vi "SVT UFF58 Write Time Waveform (1 Ch).vi"(0 "file refnum":refnum<k20>, 1 "ID lines (1-3)":T2, 2 "data precision (double-precision:1)":T1=1 items=["single-precision", "double-precision"], 5 "waveform":waveform(dbl)={"t0"=timestamp(0 s since 1904-01-01), "dt"=0.0, "Y"=[]}, 11 "error in (no error)":errorcluster) -> (4 "dup file refnum":refnum<k20>, 6 "function refnum":refnum<k20>, 15 "error out":errorcluster)   [LabVIEW 2017, in "SoundVib_UFF58.lvlib"]
doc: "Writes data to the UFF58 (universal file format) file specified by the <B>file refnum</B> input. This VI also writes the fields in records 1, 2, and 3, <B>ID lines (1-3)</B>. You can write a single time domain waveform, multiple time domain waveforms, a single real frequency spectrum, multiple real frequency spectra, a single complex frequency spectrum, multiple complex frequency spectra, or generic data to a UFF file. If a frequency spectrum is in decibels, this VI converts the spectrum to linear before writing to the UFF58 file. The default instance, SVT UFF58 Write Time Waveform (1 Ch), writes a single time domain waveform to the file specified by the <B>file refnum</B> input. Wire data to the <B>file refnum</B> input to determine the polymorphic instance to use or manually select the instance."
uses:
  <vilib>/addons/Sound and Vibration/svt_UFF58/SoundVib_UFF58.lvlib
  <vilib>/addons/Sound and Vibration/svt_UFF58/subVIs/sv_IDLines123.ctl
  <vilib>/addons/Sound and Vibration/svt_UFF58/subVIs/sv_UFF58 Data Precision.ctl
  <vilib>/addons/Sound and Vibration/svt_UFF58/subVIs/sv_UFF58 Check Data Valid (Time) (1Ch).vi
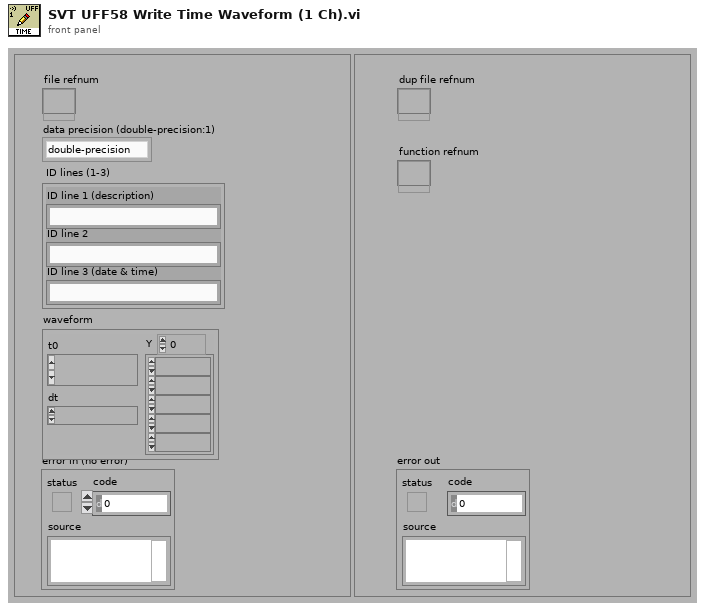
[diagram p1: front panel]
types:
  T1 = typedef "SoundVib_UFF58.lvlib/sv_UFF58 Data Precision.ctl" = u32
  T2 = typedef "SoundVib_UFF58.lvlib/sv_IDLines123.ctl" = cluster{"ID line 1 (description)":string, "ID line 2":string, "ID line 3 (date & time)":string}
  T3 = typedef "SoundVib_UFF58.lvlib/sv_UFF58 DOF.ctl" = cluster{"function type":T4, "function ID number":i32, "version number":i32, "load case ID number":i32, "response entity name":string, "response node":i32, "response direction":T5, "reference entity name":string, "reference node":i32, "reference direction":T5}
  T4 = typedef "SoundVib_UFF58.lvlib/sv_FunctionType.ctl" = enum16{"general or unknown", "time response", "auto spectrum", "cross spectrum", "frequency response function", "transmissibility", "coherence", "auto correlation", "cross correlation", "power spectral density (PSD)", "energy spectral density (ESD)", "probability density function", "spectrum", "cumulative frequency distribution", "peaks valley", "stress/cycles", "strain/cycles", "orbit", "mode indicator function", "force pattern", "partial power", "partial coherence", "eigenvalue", "eigenvector", "shock response spectrum", "finite impulse response filter", "multiple coherence", "order function", "phase compensation"}
  T5 = typedef "SoundVib_UFF58.lvlib/sv_UFF58 Response Direction.ctl" = i32
  T6 = typedef "SoundVib_UFF58.lvlib/sv_UFF58 Axis Characteristics.ctl" = cluster{"specific data type":T7, "length units exponent":i32, "force units exponent":i32, "temperature units exponent":i32, "axis label":string, "axis units label":string}
  T7 = typedef "SoundVib_UFF58.lvlib/sv_UFF58 Specific Datatype.ctl" = u16
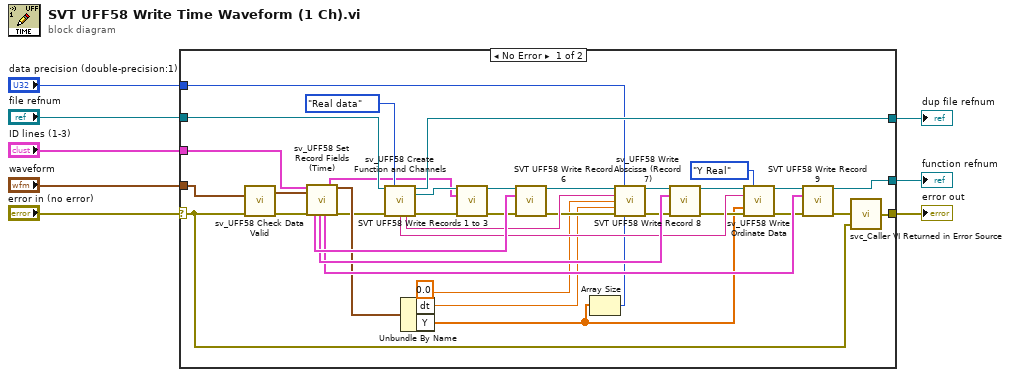
[diagram p0: block diagram]
diagram:
  n1 = case shown="No Error" "error in (no error)" {
    selector: "error in (no error)" -> [w13 w47]
    tunnel: [w14 w47] -> w8
    tunnel: "ID lines (1-3)" -> [w39 _]
    tunnel: [w23 w46] -> w6
    tunnel: "file refnum" -> [w35 w46]
    tunnel: "waveform" -> [w11 _]
    tunnel: [w24 _] -> w2
    tunnel: "data precision (double-precision:1)" -> [w9 _]
    frame No Error {
      n2 = call-poly <vilib>:"sv_UFF58 Check Data Valid.vi"("waveform"=w11, "error in (no error)"=w13) -> ("dup waveform"=w19:waveform(dbl), "error out"=w20:errorcluster)  [unwired: 12 in]
      n3 = call <vilib>:"sv_UFF58 Set Record Fields (Time).vi"("ID lines (1-3)"=w39, "waveform"=w19, "error in (no error)"=w20) -> ("DOF identification (record 6)"=w45:T3, "abscissa data characteristics (record 8)"=w44:T6, "ordinate numerator data characteristics (record 9)"=w43:T6, "ID lines (1-3) out"=w12:T2, "dup waveform"=w40:waveform(dbl), "error out"=w22:errorcluster)  [unwired: 11 in]
      n4 = call <vilib>:"sv_UFF58 Create Function and Channels.vi"("file refnum"=w35, "real or complex data?"=enum16{"Real data", "Complex data"}."Real data", "error in (no error)"=w22) -> ("dup file refnum"=w23:refnum<k20>, "function refnum"=w34:refnum<k20>, "ordinate numerator channel name"=w42:string, "abscissa channel name"=w41:string, "error out"=w33:errorcluster)  [unwired: 6 in, 2 out]
      n5 = Unbundle By Name(w40) -> ("dt"=w28:dbl, "Y"=w17:dbl[])
      n6 = call <vilib>:"SVT UFF58 Write Records 1 to 3.vi"("function refnum"=w34, "ID lines (1-3)"=w12, "error in (no error)"=w33) -> ("dup function refnum"=w38:refnum<k20>, "error out"=w37:errorcluster)  [unwired: 11 in]
      n7 = call <vilib>:"SVT UFF58 Write Record 6.vi"("function refnum"=w38, "DOF identification"=w45, "error in (no error)"=w37) -> ("dup function refnum"=w26:refnum<k20>, "error out"=w32:errorcluster)  [unwired: 11 in]
      n8 = Array Size(array=w17) -> (size(s)=w16:i32)
      n9 = call <vilib>:"sv_UFF58 Write Abscissa (Record 7).vi"("function refnum"=w26, "data precision (double-precision:1)"=w9, "Name"=w41, "x0"=0.0 ("dt"), "dx"=w28, "error in (no error)"=w32, "channel length"=w16) -> ("dup function refnum"=w27:refnum<k20>, "error out"=w36:errorcluster)  [unwired: 7 in]
      n10 = call <vilib>:"SVT UFF58 Write Record 8.vi"("function refnum"=w27, "abscissa data characteristics"=w44, "error in (no error)"=w36) -> ("dup function refnum"=w25:refnum<k20>, "error out"=w30:errorcluster)  [unwired: 11 in]
      n11 = call <vilib>:"sv_UFF58 Write Ordinate Data.vi"("function refnum"=w25, "channel to write"=enum16{"X", "Y Real", "Y Imaginary"}."Y Real", "ordinate channel name"=w42, "ordinate data"=w17, "error in (no error)"=w30) -> ("dup function refnum"=w29:refnum<k20>, "error out"=w31:errorcluster)  [unwired: 9 in]
      n12 = call <vilib>:"SVT UFF58 Write Record 9.vi"("function refnum"=w29, "ordinate data characteristics"=w43, "error in (no error)"=w31) -> ("dup function refnum"=w24:refnum<k20>, "error out"=w15:errorcluster)  [unwired: 11 in]
      n13 = call <vilib>:"svc_Caller VI Returned in Error Source.vi"("warning input to caller"=w13, "error in (no error)"=w15) -> ("error out"=w14:errorcluster)  [unwired: 3 in]
    }
    frame Error {
    }
  }
  "dup file refnum" <- w6
  "error out" <- w8
  "function refnum" <- w2
